vi "On Settings Modified.vi"(7 "Action":T1, 11 "UI Data in":refnum<class "Settings UI.lvclass">) -> (3 "UI Data out":refnum<class "Settings UI.lvclass">)   [LabVIEW 2020, in "Output Sequencer.lvlib" / "Settings UI.lvclass"]
uses:
  Settings UI.lvclass
  Types/Settings UI Action.ctl
  Settings UI.lvclass/Settings UI.ctl
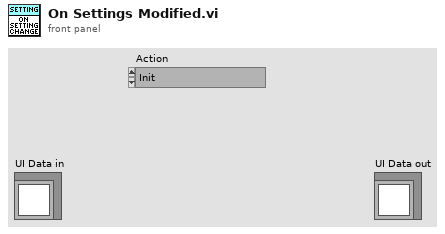
[diagram p1: front panel]
types:
  T1 = typedef "Output Sequencer.lvlib/Settings UI.lvclass/Settings UI Action.ctl" = enum16{"Init", "Timeout", "Tree Change", "Tree Mouse Down", "Value Change", "Expand All", "Show Overview", "Collapse All", "Insert Above", "Insert Below", "Remove Step", "Move Up", "Move Down", "Drag Starting", "Drag Over", "Drop", "Drag Ended", "Import"}
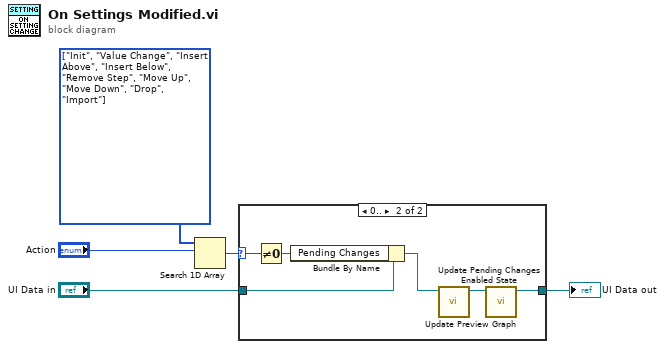
[diagram p0: block diagram]
diagram:
  w4 = T1[] [enum."Init", enum."Value Change", enum."Insert Above", enum."Insert Below", enum."Remove Step", enum."Move Up", enum."Move Down", enum."Drop", enum."Import"] items=["Init", "Timeout", "Tree Change", "Tree Mouse Down", "Value Change", "Expand All", "Show Overview", "Collapse All", "Insert Above", "Insert Below", "Remove Step", "Move Up", "Move Down", "Drag Starting", "Drag Over", "Drop", "Drag Ended", "Import"]
  n1 = Search 1D Array(1D array=w4, element="Action") -> (index of element=w3:i32)  [unwired: 1 in]
  n2 = case shown="0.." w3 {
    selector: w3 -> [_ w12]
    tunnel: "UI Data in" -> [w6 w11]
    tunnel: [w6 w10] -> w2
    frame Default {
    }
    frame 0.. {
      n3 = Not Equal To 0?(x=w12) -> (x != 0?=w8:bool)
      n4 = Bundle By Name(cluster=w11, "Pending Changes"=w8) -> (w7:refnum<class "Settings UI.lvclass">)
      n5 = call "Update Pending Changes Enabled State.vi"("UI Data in"=w7) -> ("UI Data out"=w9:refnum<class "Settings UI.lvclass">)  [unwired: 10 in]
      n6 = call "Update Preview Graph.vi"("UI Data in"=w9) -> ("UI Data out"=w10:refnum<class "Settings UI.lvclass">)  [unwired: 10 in]
    }
  }
  "UI Data out" <- w2
